vi "Optical Flow Obstacle Avoidance.vi"() -> ()   [LabVIEW 2015]
doc: "This example shows use the Horn Schunck and Lucas Kanade methods to compute dense optical (motion) flow information in a sequence of images. The VI reads the frames and computes the optical flow between consecutive frames."
uses:
  <vilib>/imath/engines/lvmath2/RunTimeEngine/Managers/WorkSpace/UID Generator.vi
  <vilib>/imath/engines/lvmath2/RunTimeEngine/BuiltInFunctions/curl/NIMS_[2o]_curl(M,M).vi
  <vilib>/imath/engines/lvmath2/RunTimeEngine/RunTimeType/NIMS_RunTimeType_From StrictType (excl LVString).vi
  <instcachedir>/0/NIMS_RunTimeType_From StrictType (excl LVString)_EB1C38A9BC5048DA9ABDA8F781E54D21.lvgen/NIMS_RunTimeType_From StrictType (excl LVString)_EB1C38A9BC5048DA9ABDA8F781E54D21_000.vi
  <vilib>/imath/engines/lvmath2/RunTimeEngine/ErrorHandling/NIMS_Error From Error Code.vi
  <vilib>/imath/engines/lvmath2/RunTimeEngine/LocalVariableDefStatement/MC_LocalVariableDefStatement_Display.vi
  <vilib>/imath/engines/lvmath2/RunTimeEngine/BuiltInFunctions/divergence/NIMS_divergence(M,M).vi
  <vilib>/imath/engines/lvmath2/RunTimeEngine/Managers/SymbolTable/Clear UID.vi
  <vilib>/imath/engines/lvmath2/RunTimeEngine/NodeEndStatement/NIMS_NodeEndStatement_Output.vi
  <instcachedir>/0/NIMS_NodeEndStatement_Output_53EC0D466D134D7ABD903AC30B43404B.lvgen/NIMS_NodeEndStatement_Output_53EC0D466D134D7ABD903AC30B43404B_002.vi
  <vilib>/imath/engines/lvmath2/RunTimeEngine/ErrorHandling/NIMS_Finalize Error.vi
  <vilib>/vision/NI_Vision_Development_Module.lvlib
  <vilib>/imath/engines/lvmath2/RunTimeEngine/Managers/SymbolTable/NIMS_WorkSpace.lvlib
panel:
  in  "Window Size (15x15)":cluster{"Size X":i32, "Size Y":i32}={"Size X"=7, "Size Y"=7}
  in  "Curl threshold":dbl=10.0 format="%#_13g"
  out "Image":T1(plugin-control)
  in  "Size & Order # 2":T2={"X Size"=3, "Y Size"=3, "Order #"=4}
  in  "Size & Order #":T2={"X Size"=3, "Y Size"=3, "Order #"=4}
  out "fitlered curl":dbl[][](graph)
  in  "Video Sequence Folder Path":path
  in  "Delay (s.)":dbl(slide)=0.25 scale=0.0..1.5
  out "Progress Bar":i32(slide) max=783 scale=-1.0..783.0
  in  "Stop":bool
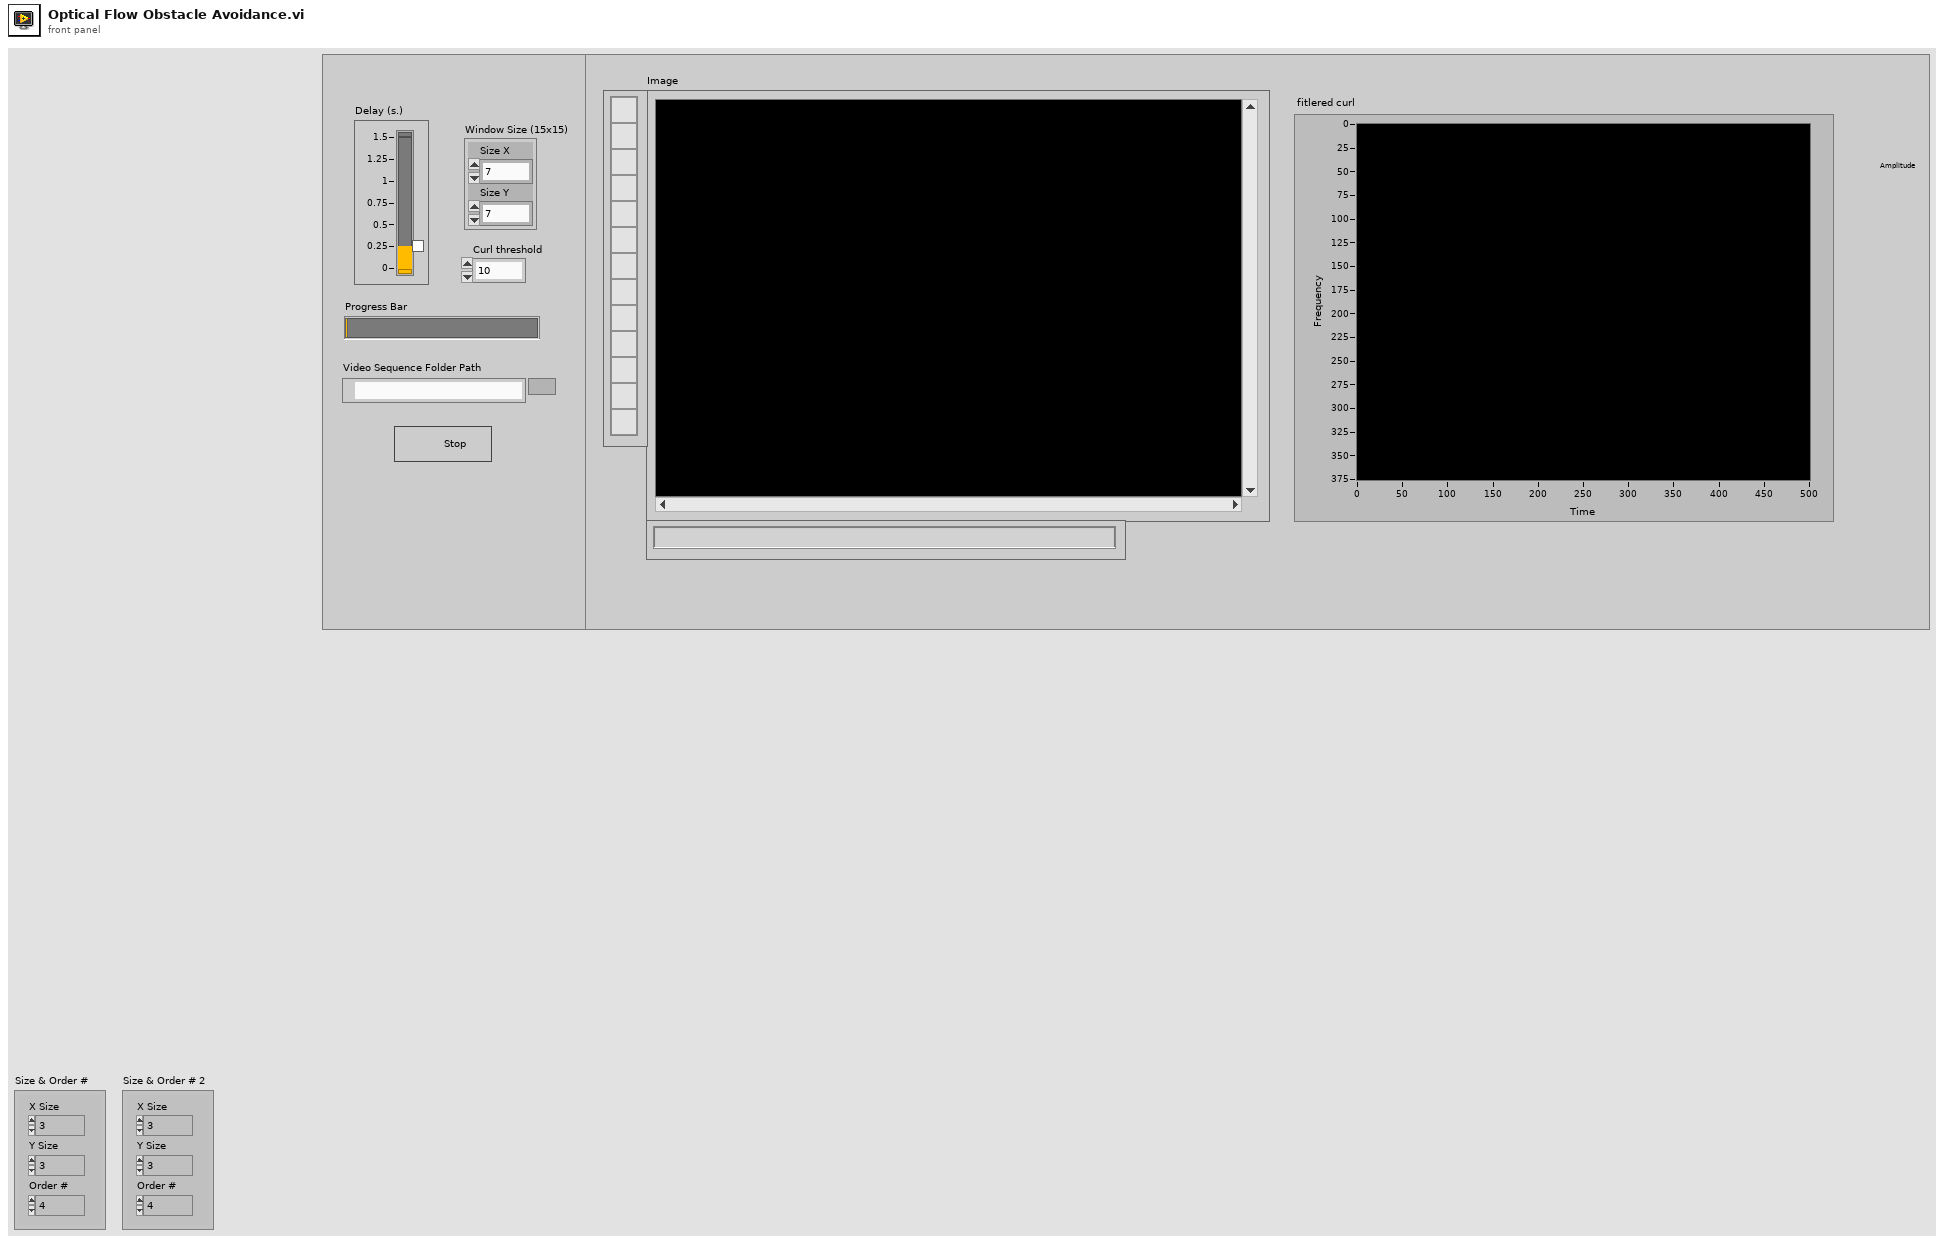
[diagram p1: front panel]
types:
  T1 = typedef "IMAQ Image.ctl" = refnum<image>
  T2 = cluster{"X Size":i32, "Y Size":i32, "Order #":i32}
  T3 = typedef "Image Type" = u32
  T4 = cluster{"Global Rectangle":i32[], "Contours":cluster{"Contour Type":u32, "ROI Type":u32, "Points":i32[]}[]}
  T5 = cluster{"Left":i32, "Top":i32, "Right":i32, "Bottom":i32}
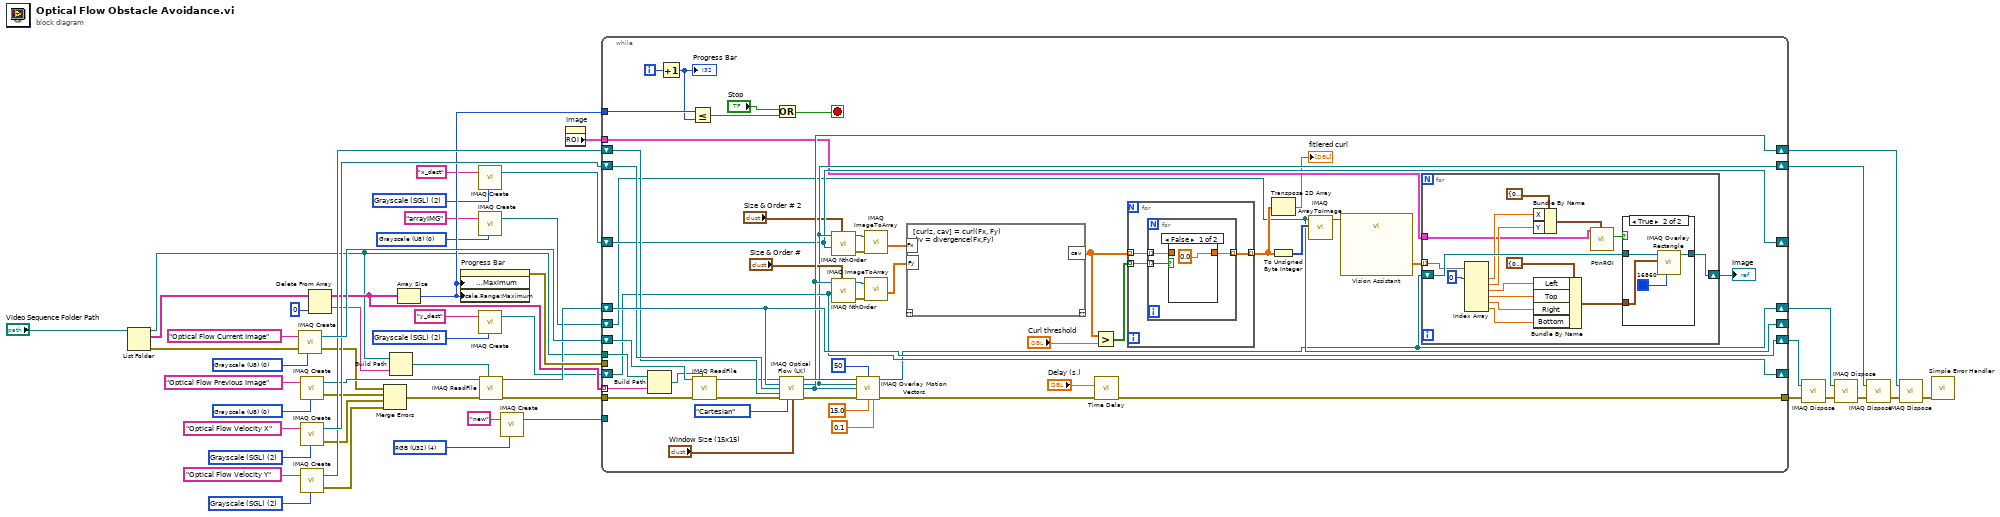
[diagram p0: block diagram]
diagram:
  w5 = T3 0 items=["Grayscale (U8)", "Grayscale (I16)", "Grayscale (SGL)", "Complex (CSG)", "RGB (U32)", "HSL (U32)", "RGB (U64)", "Grayscale (U16)"] ("Image Type")
  w7 = T3 4 items=["Grayscale (U8)", "Grayscale (I16)", "Grayscale (SGL)", "Complex (CSG)", "RGB (U32)", "HSL (U32)", "RGB (U64)", "Grayscale (U16)"] ("Image Type")
  w9 = T3 2 items=["Grayscale (U8)", "Grayscale (I16)", "Grayscale (SGL)", "Complex (CSG)", "RGB (U32)", "HSL (U32)", "RGB (U64)", "Grayscale (U16)"] ("Image Type")
  w10 = T3 2 items=["Grayscale (U8)", "Grayscale (I16)", "Grayscale (SGL)", "Complex (CSG)", "RGB (U32)", "HSL (U32)", "RGB (U64)", "Grayscale (U16)"] ("Image Type")
  w27 = T3 2 items=["Grayscale (U8)", "Grayscale (I16)", "Grayscale (SGL)", "Complex (CSG)", "RGB (U32)", "HSL (U32)", "RGB (U64)", "Grayscale (U16)"] ("Image Type")
  w28 = T3 0 items=["Grayscale (U8)", "Grayscale (I16)", "Grayscale (SGL)", "Complex (CSG)", "RGB (U32)", "HSL (U32)", "RGB (U64)", "Grayscale (U16)"] ("Image Type")
  w42 = T3 0 items=["Grayscale (U8)", "Grayscale (I16)", "Grayscale (SGL)", "Complex (CSG)", "RGB (U32)", "HSL (U32)", "RGB (U64)", "Grayscale (U16)"] ("Image Type")
  w44 = T3 2 items=["Grayscale (U8)", "Grayscale (I16)", "Grayscale (SGL)", "Complex (CSG)", "RGB (U32)", "HSL (U32)", "RGB (U64)", "Grayscale (U16)"] ("Image Type")
  n1 = List Folder(path="Video Sequence Folder Path") -> (path out=w31:path, filenames=w35:string[], error out=w26:errorcluster)  [unwired: 1 in, 3 out]
  n2 = call "IMAQ Create"("Image Name"="Optical Flow Current Image", "Image Type"=w42, "error in (no error)"=w26) -> ("New Image"=w50:T1, "error out"=w25:errorcluster)  [unwired: 1 in, 1 out]
  n3 = call "IMAQ Create"("Image Name"="Optical Flow Previous Image", "Image Type"=w28) -> ("New Image"=w37:T1, "error out"=w23:errorcluster)  [unwired: 2 in, 1 out]
  n4 = call "IMAQ Create"("Image Name"="Optical Flow Velocity X", "Image Type"=w44) -> ("New Image"=w47:T1, "error out"=w22:errorcluster)  [unwired: 2 in, 1 out]
  n5 = call "IMAQ Create"("Image Name"="Optical Flow Velocity Y", "Image Type"=w27) -> ("New Image"=w43:T1, "error out"=w24:errorcluster)  [unwired: 2 in, 1 out]
  n6 = Delete From Array(array=w35, index=0) -> (deleted portion=w30:string, array with subset deleted=w32:string[])  [unwired: 1 in]
  n7 = Merge Errors(w25, w23, w22, w24) -> (w21:errorcluster)
  n8 = Build Path(base path=w31, name or relative path=w30) -> (appended path=w29:path)
  n9 = Array Size(array=w32) -> (size(s)=w33:i32)
  n10 = property on="Progress Bar" class="Slide (strict)"("Data Entry Limits:Maximum"=w33, "Scale.Range:Maximum"=w33) -> (error out=w49:errorcluster)  [unwired: 2 in, 1 out]
  n11 = call "IMAQ Create"("Image Name"="x_dest", "Image Type"=w10) -> ("New Image"=w11:T1)  [unwired: 2 in, 2 out]
  n12 = call "IMAQ Create"("Image Name"="arrayIMG", "Image Type"=w5) -> ("New Image"=w3:T1)  [unwired: 2 in, 2 out]
  n13 = call "IMAQ Create"("Image Name"="y_dest", "Image Type"=w9) -> ("New Image"=w13:T1)  [unwired: 2 in, 2 out]
  n14 = call "IMAQ ReadFile"("File Path"=w29, "error in (no error)"=w21, "Image"=w37) -> ("error out"=w1:errorcluster, "Image Out"=w36:T1)  [unwired: 2 in, 5 out]
  n15 = call "IMAQ Create"("Image Name"="new", "Image Type"=w7) -> ("New Image"=w6:T1)  [unwired: 2 in, 2 out]
  n16 = property on="Image" class="ImageControl"() -> ("ROI"=w2:T4)  [unwired: 2 in, 2 out]
  n17 = while {
    tunnel: [w92] -> w20
    tunnel: w33 -> [w100]
    tunnel: w49 -> [_]
    shift-right: [w71] -> w40
    shift-left: w47 -> [w98]
    shift-right: [w77] -> w39
    shift-left: w43 -> [w97]
    shift-right: [w56] -> w38
    shift-left: w36 -> [w99]
    tunnel: w31 -> [w95]
    tunnel: w32 -> [w94] mode=indexing
    shift-right: [w99] -> w41
    shift-left: w50 -> [w101]
    shift-right: [w74] -> _
    shift-left: w13 -> [w74]
    shift-right: [w68] -> _
    shift-left: w11 -> [w68]
    tunnel: w6 -> [_]
    shift-right: [w59] -> _
    shift-left: w3 -> [w59]
    tunnel: w2 -> [w57]
    tunnel: w1 -> [w54]
    i -> [w93]
    stop <- w79 stop-if-true
    n18 = Build Path(base path=w95, name or relative path=w94) -> (appended path=w83:path)
    n19 = Increment(x=w93) -> (x+1=w96:i32)
    "Progress Bar" <- w96
    n20 = Less Or Equal?(x=w100, y=w96) -> (x <= y?=w90:bool)
    n21 = call "IMAQ ReadFile"("File Path"=w83, "error in (no error)"=w54, "Image"=w101) -> ("error out"=w88:errorcluster, "Image Out"=w87:T1)  [unwired: 2 in, 5 out]
    n22 = Or(x="Stop", y=w90) -> (x .or. y?=w79:bool)
    n23 = call "IMAQ Optical Flow (LK)"("Current Frame"=w87, "Previous Frame"=w99, "Velocity Component 1 In"=w98, "Velocity Component 2 In"=w97, "error in (no error)"=w88, "Velocity Representation"=enum16{"Cartesian", "Polar"}."Cartesian", "Window Size (15x15)"="Window Size (15x15)") -> ("Current Frame Out (dup)"=w85:T1, "Velocity Component 1 Out"=w71:T1, "Velocity Component 2 Out"=w77:T1, "error out"=w86:errorcluster)  [unwired: 1 in, 4 out]
    n24 = call "IMAQ NthOrder"("Image Src"=w71, "Size & Order #"="Size & Order # 2", "Image Dst"=w68) -> ("Image Dst Out"=w70:T1, "error out"=w69:errorcluster)  [unwired: 4 in]
    n25 = call "IMAQ NthOrder"("Image Src"=w77, "Size & Order #"="Size & Order #", "Image Dst"=w74) -> ("Image Dst Out"=w76:T1, "error out"=w75:errorcluster)  [unwired: 4 in]
    n26 = call "IMAQ Overlay Motion Vectors"("Image"=w85, "Step Size"=50, "Velocity Component 1"=w71, "Velocity Component 2"=w77, "error in (no error)"=w86, "Scale"=15.0, "Threshold"=0.1) -> ("Image Out"=w56:T1, "error out"=w72:errorcluster)  [unwired: 3 in, 4 out]
    n27 = call "IMAQ ImageToArray"("error in (no error)"=w69, "Image"=w70) -> ("Image Pixels (Float)"=w66:sgl[][])  [unwired: 2 in, 4 out]
    n28 = call "IMAQ ImageToArray"("error in (no error)"=w75, "Image"=w76) -> ("Image Pixels (Float)"=w78:sgl[][])  [unwired: 2 in, 4 out]
    n29 = mathscript code="[curlz, cav] = curl(Fx, Fy)\ndiv = divergence(Fx,Fy)"("Fx"=w66, "Fy"=w78) -> ("cav"=w53:dbl[][])  [unwired: 1 in, 1 out]
    n30 = Greater?(x=w53, y="Curl threshold") -> (0:w64:bool[][])
    n31 = call "Time Delay"("error in (no error)"=w72, "Delay Time (s)"="Delay (s.)") -> ("error out"=w92:errorcluster)  [unwired: 9 in]
    n32 = for {
      tunnel: w64 -> [w125] mode=indexing
      tunnel: w53 -> [w124] mode=indexing
      tunnel: [w123] -> w62 mode=indexing
      n33 = for {
        tunnel: w125 -> [w128] mode=indexing
        tunnel: w124 -> [w127] mode=indexing
        tunnel: [w126] -> w123 mode=indexing
        n34 = case shown="False" w128 {
          tunnel: w127 -> [_ w130]
          tunnel: [sgl 0.0 w130] -> w126
          frame False {
          }
          frame True {
          }
        }
      }
    }
    n35 = To Unsigned Byte Integer(number=w62) -> (unsigned 8bit integer=w61:u8[][])
    n36 = Transpose 2D Array(2D array=w62) -> (transposed array=→"fitlered curl":dbl[][])
    n37 = call "IMAQ ArrayToImage"("Image Pixels (U8)"=w61, "Image"=w59) -> ("Image Out"=w60:T1)  [unwired: 8 in, 1 out]
    n38 = call "Vision Assistant"("Image In"=w60) -> ("Particle Measurements (Pixels) (Particle Analysis 1)"=w58:dbl[][])  [unwired: 24 in, 2 out]
    n39 = for {
      tunnel: w57 -> [w110]
      shift-right: [w116] -> w55
      shift-left: w56 -> [w117]
      tunnel: w58 -> [w114] mode=indexing
      n40 = Index Array(array=w114, index #1=0 ("index")) -> (element #1=w112:dbl, element #2=w111:dbl, element #3=w106:dbl, element #4=w105:dbl, element #5=w104:dbl, element #6=w103:dbl)  [unwired: 5 in]
      n41 = Bundle By Name(cluster=cluster{"X":dbl, "Y":dbl} {"X"=0.0, "Y"=0.0} ("Point"), "X"=w112, "Y"=w111) -> (w108:cluster{"X":dbl, "Y":dbl})
      n42 = Bundle By Name(cluster=T5 {"Left"=0, "Top"=0, "Right"=0, "Bottom"=0} ("Rectangle"), "Left"=w106, "Top"=w105, "Right"=w104, "Bottom"=w103) -> (w102:T5)
      n43 = call "PtInROI.vi"("Point"=w108, "ROI Descriptor In"=w110) -> ("IsInside"=w109:bool)  [unwired: 8 in, 1 out]
      n44 = case shown="True" w109 {
        tunnel: w117 -> [w118 w122]
        tunnel: [w118 w119] -> w116
        tunnel: w102 -> [_ w120]
        frame False {
        }
        frame True {
          n45 = call "IMAQ Overlay Rectangle"("Color"=u32 16860 ("color(green)"), "Rectangle"=w120, "Image"=w122) -> ("Image Out"=w119:T1)  [unwired: 7 in, 1 out]
        }
      }
    }
    "Image" <- w55
  }
  n46 = call "IMAQ Dispose"("Image"=w41, "error in (no error)"=w20) -> ("error out"=w19:errorcluster)  [unwired: 1 in, 3 out]
  n47 = call "IMAQ Dispose"("Image"=w38, "error in (no error)"=w19) -> ("error out"=w18:errorcluster)  [unwired: 1 in, 3 out]
  n48 = call "IMAQ Dispose"("Image"=w40, "error in (no error)"=w18) -> ("error out"=w17:errorcluster)  [unwired: 1 in, 3 out]
  n49 = call "IMAQ Dispose"("Image"=w39, "error in (no error)"=w17) -> ("error out"=w16:errorcluster)  [unwired: 1 in, 3 out]
  n50 = call <vilib>:"Simple Error Handler.vi"("error in (no error)"=w16) -> ()  [unwired: 1 in, 8 out]
